vi "Set ID.vi"(10 "ID":string, 11 "IConnection in":refnum<class "IConnection.lvclass">) -> (3 "IConnection out":refnum<class "IConnection.lvclass">)   [LabVIEW 2020, in "Connection Reference.lvlib" / "IConnection.lvclass"]
uses:
  <vilib>/gpm_packages/@cs/Network-interface/Source/Connection Reference/IConnection/IConnection.lvclass
  <vilib>/gpm_packages/@cs/Network-interface/Source/Connection Reference/IConnection/IConnection.lvclass/IConnection.ctl
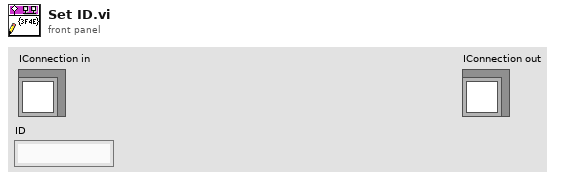
[diagram p1: front panel]
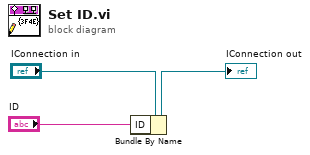
[diagram p0: block diagram]
diagram:
  n1 = Bundle By Name(cluster="IConnection in", "ID"="ID") -> (→"IConnection out":refnum<class "IConnection.lvclass">)
